vi "parseDisplacementResponse.vi"(8 "error in (no error)":errorcluster, 10 "DynamicFrameParser":refnum<class "DynamicFrameParser.lvclass">, 11 "MDILC in":refnum<class "MDILC.lvclass">) -> (0 "error out":errorcluster, 3 "MDILC out":refnum<class "MDILC.lvclass">)   [LabVIEW 2016, in "RTMDILC.lvlib" / "MDILC.lvclass"]
uses:
  MDILC.lvclass
  Common_RT_Modbus/DynamicFrameParser/DynamicFrameParser.lvclass
  Common_RT_Modbus/DataTypes/ExceptionCodes.ctl
  MDILC.lvclass/MDILC.ctl
  Common_RT_Modbus/RTModbus.lvlib
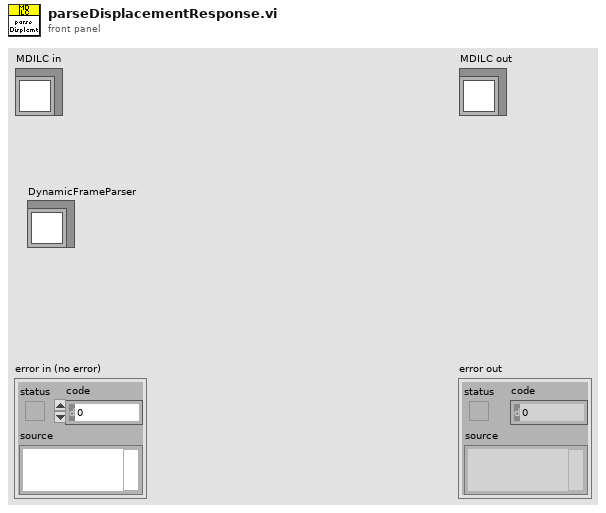
[diagram p1: front panel]
types:
  T1 = typedef "RTModbus.lvlib/ExceptionCodes.ctl" = u16
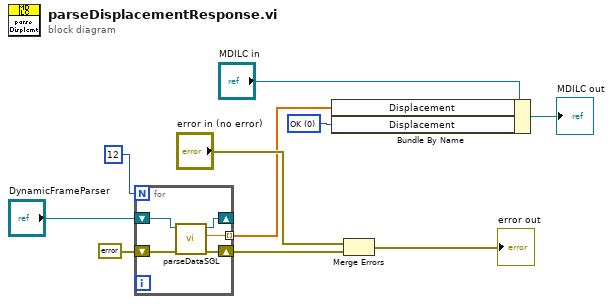
[diagram p0: block diagram]
diagram:
  w5 = T1 0 items=["OK", "IllegalFunction", "IllegalDataAddress", "IllegalDataValue", "SlaveDeviceFailure", "Acknowledge", "SlaveDeviceBusy", "NegativeAcknowledge", "MemoryParityError", "GatewayPathUnavailable", "GatewayTargetDeviceFailedToRespond"] ("MTData.MTResponses.Temperature")
  n1 = for {
    N: 12 -> [_]
    shift-right: [w14] -> _
    shift-left: "DynamicFrameParser" -> [w15]
    tunnel: [w13] -> w4 mode=indexing
    shift-right: [w12] -> w1
    shift-left: errorcluster {"status"=FALSE, "code"=0, "source"=""} ("error out") -> [w11]
    n2 = call "parseDataSGL.vi"("error in (no error)"=w11, "FrameParser in"=w15) -> ("error out"=w12:errorcluster, "Data"=w13:sgl, "FrameParser out"=w14:refnum<class "DynamicFrameParser.lvclass">)  [unwired: 7 in]
  }
  n3 = Bundle By Name(cluster="MDILC in", "Displacement"=w4, "Displacement"=w5) -> (→"MDILC out":refnum<class "MDILC.lvclass">)
  n4 = Merge Errors("error in (no error)", w1) -> (→"error out":errorcluster)
